vi "Add Port.vi"(8 "error in":errorcluster, 9 "direction":T1, 10 "port number":u16, 11 "custom device ref":T2 format="%.0x") -> (0 "error out":errorcluster, 2 "port ref out":T2 format="%.0x", 3 "custom device ref out":T2 format="%.0x")   [LabVIEW 2020, in "Ballard ARINC 429 Scripting.lvlib"]
doc: "Based on the specified <b>direction</b>, adds the specified <b>port</b> to the system definition. Receive (Rx) ports are added to the Ports>>Incoming subsection. Transmit (Tx) ports are added to the Ports>>Outgoing subsection."
uses:
  <vilib>/addons/VeriStand Custom Device Scripting APIs/Ballard ARINC 429/Custom Device Support/Scripting/Ballard/Ballard ARINC 429 Scripting.lvlib
  <vilib>/NI VeriStand/Custom Device API/Custom Device Item Ref.ctl
  <vilib>/addons/VeriStand Custom Device Scripting APIs/Ballard ARINC 429/Custom Device Support/Shared/Direction.ctl
  <vilib>/addons/VeriStand Custom Device Scripting APIs/Ballard ARINC 429/Custom Device Support/Scripting/Ballard/Constants.vi
  <vilib>/NI VeriStand/Custom Device Tools/Custom Device Utility Library/NI VeriStand - Search for Item by GUID.vi
  <vilib>/NI VeriStand/Custom Device API/Custom Device API.lvlib
  <vilib>/NI VeriStand/Custom Device Tools/Custom Device Utility Library/Custom Device Utility Library.lvlib
  <vilib>/addons/VeriStand Custom Device Scripting APIs/Ballard ARINC 429/Custom Device Support/Scripting/ARINC 429/ARINC 429 Scripting.lvlib
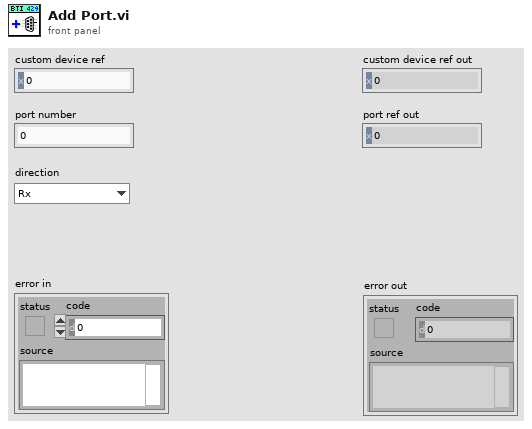
[diagram p1: front panel]
types:
  T1 = typedef "Direction.ctl" = enum16{"Rx", "Tx"}
  T2 = typedef "Custom Device API.lvlib/Custom Device Item Ref.ctl" = u64
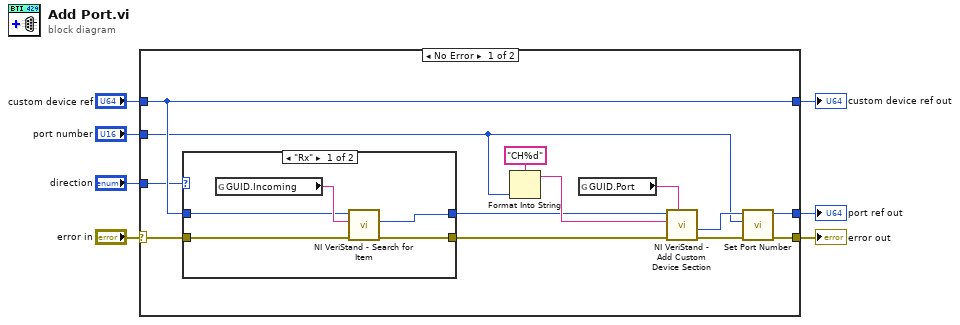
[diagram p0: block diagram]
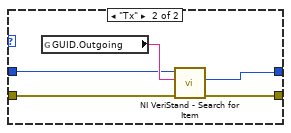
[diagram p2: hidden frame]
diagram:
  n1 = case shown="No Error" "error in" {
    selector: "error in" -> [w17 w32]
    tunnel: "custom device ref" -> [w14 w31]
    tunnel: [w11 w32] -> w6
    tunnel: [w9 _] -> w5
    tunnel: "port number" -> [w8 _]
    tunnel: [w14 w31] -> w2
    tunnel: "direction" -> [w13 _]
    frame No Error {
      n2 = case shown="\"Rx\"" w13 {
        tunnel: w14 -> [w22 w28]
        tunnel: [w23 w26] -> w15
        tunnel: w17 -> [w21 w29]
        tunnel: [w24 w27] -> w16
        frame "Rx" {
          n3 = global read "Constants.vi" "GUID.Incoming"() -> (w25:string)
          n4 = call-poly <vilib>:"NI VeriStand - Search for Item.vi"("error in"=w21, "Item GUID"=w25, "Section Ref in"=w22) -> ("error out"=w24:errorcluster, "Item Ref"=w23:T2)  [unwired: 5 in, 2 out]
        }
        frame "Tx" {
          n5 = global read "Constants.vi" "GUID.Outgoing"() -> (w30:string)
          n6 = call-poly <vilib>:"NI VeriStand - Search for Item.vi"("error in"=w29, "Item GUID"=w30, "Section Ref in"=w28) -> ("error out"=w27:errorcluster, "Item Ref"=w26:T2)  [unwired: 5 in, 2 out]
        }
      }
      n7 = Format Into String(format string="CH%d", w8) -> (resulting string=w18:string)  [unwired: 2 in, 1 out]
      n8 = global read "Constants.vi" "GUID.Port"() -> (w20:string)
      n9 = call <vilib>:"NI VeriStand - Add Custom Device Section.vi"("GUID (Default Section)"=w20, "error in (no error)"=w16, "Section Name"=w18, "Parent Ref in"=w15) -> ("error out"=w12:errorcluster, "Section Ptr"=w10:T2)  [unwired: 4 in, 2 out]
      n10 = call <vilib>:"Set Port Number.vi"("error in"=w12, "port number"=w8, "port ref in"=w10) -> ("error out"=w11:errorcluster, "port ref out"=w9:T2)  [unwired: 7 in]
    }
    frame Error {
    }
  }
  "error out" <- w6
  "port ref out" <- w5
  "custom device ref out" <- w2
